vi "DataFileNode_Entry_V3.vi"(8 "error in (no error)":errorcluster, 10 "remaining elements":T1[](array[typedef]), 11 "Byte Stream File in":refnum<file>) -> (0 "error out":errorcluster, 3 "Byte Stream File out":refnum<file>)   [LabVIEW 2019]
uses:
  Controls/QueueDataControl_V3.ctl
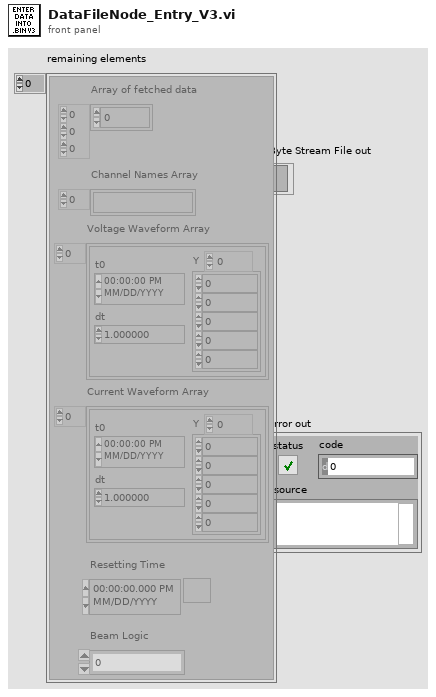
[diagram p1: front panel]
types:
  T1 = typedef "QueueDataControl_V3.ctl" = cluster{"Array of fetched data":dbl[][][], "Channel Names Array":string[], "Voltage Waveform Array":waveform(dbl)[], "Current Waveform Array":waveform(dbl)[], "Resetting Time":timestamp, "Beam Logic":dbl}
  T2 = enum16{"big-endian, network order", "native, host order", "little-endian"}
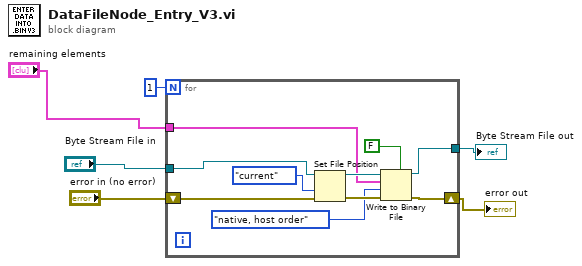
[diagram p0: block diagram]
diagram:
  n1 = for {
    N: 1 -> [_]
    tunnel: "remaining elements" -> [w10]
    shift-right: [w12] -> w5
    shift-left: "error in (no error)" -> [w13]
    tunnel: "Byte Stream File in" -> [w8]
    tunnel: [w7] -> w3
    n2 = Set File Position(refnum=w8, from (0:start)=enum16{"start", "end", "current"}."current", error in=w13) -> (refnum out=w15:refnum<file>, error out=w14:errorcluster)  [unwired: 1 in]
    n3 = Write to Binary File(file (use dialog)=w15, data=w10, error in=w14, 5:FALSE ("prepend array or string size? (T)"), 9:T2."native, host order" ("byte order (0:big-endian, network order)")) -> (refnum out=w7:refnum<file>, error out=w12:errorcluster)  [unwired: 1 in, 1 out]
  }
  "error out" <- w5
  "Byte Stream File out" <- w3
